vi "Pre-Process Module.vi"(5 "Start Acquire?":bool=TRUE, 6 "Action":string, 7 "Save":bool, 8 "error in":errorcluster, 9 "#pixels to save":i32=200, 10 "start pixel":i32, 11 "#A-lines per B-line":i32=2048) -> (0 "Error Out":errorcluster, 1 "Exit?":bool, 2 "# elements in data queue":i32)   [LabVIEW 2018]
uses:
  Controls/Queue Manager Actions.ctl
  Controls/QueueNames.ctl
  Controls/MessagePacket.ctl
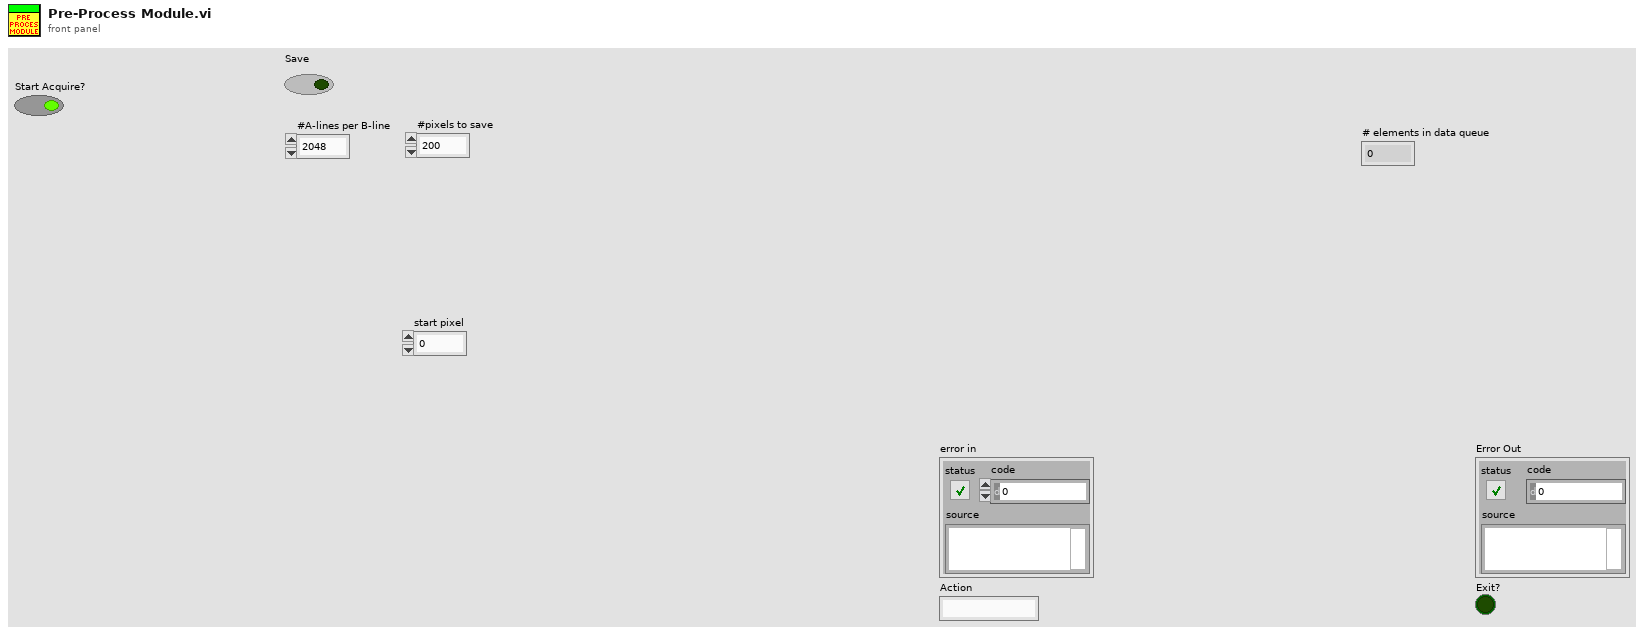
[diagram p1: front panel]
types:
  T1 = typedef "Queue Manager Actions.ctl" = enum16{"Init", "Enqueue", "Enqueue All", "Preview Queue", "Dequeue", "Get Status", "Flush Queue", "Flush All Queues", "Release All Queues", "Release Queue", "Enqueue at Opposite End"}
  T2 = typedef "MessagePacket.ctl" = cluster{"Message":string, "Parameter":variant}
  T3 = typedef "QueueNames.ctl" = enum16{"Main GUI", "Main Scan Processor", "Main Processing", "Main Saving", "Main Display", "Main Table Stage GUI", "Main Table Stage Proc.", "Scan Engine", "Vibratome GUI", "Vibratome Processor", "Slice Engine"}
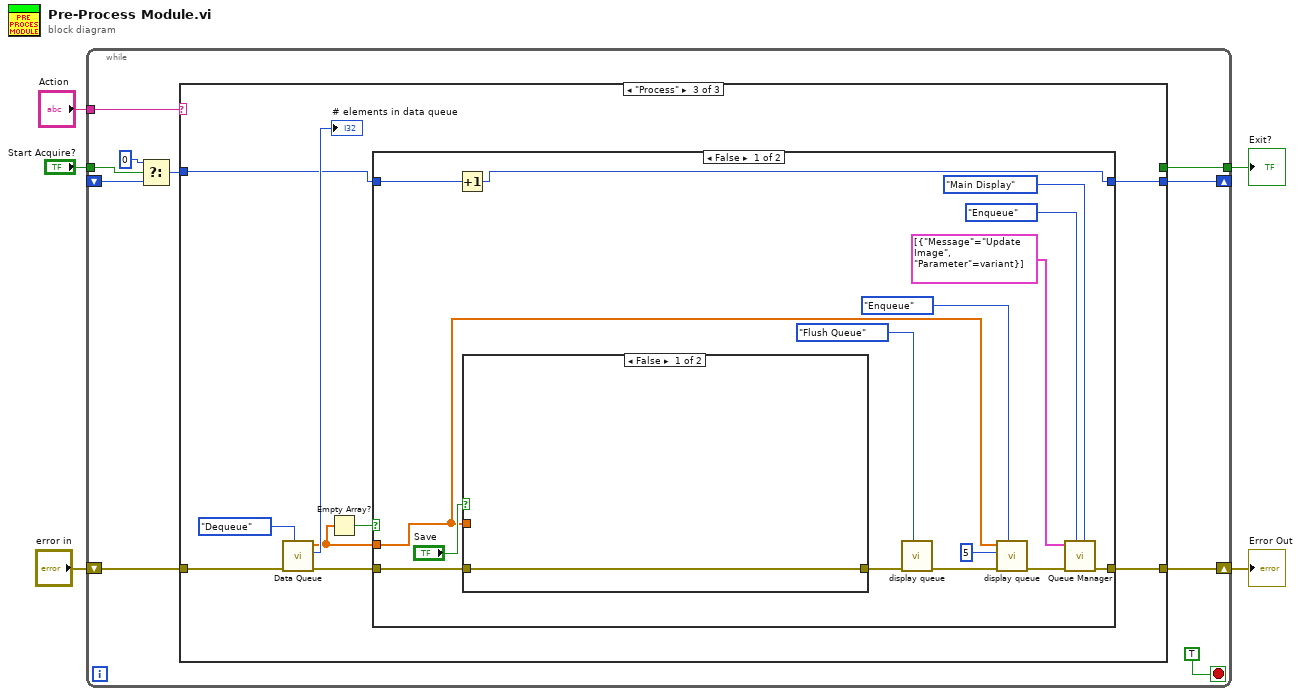
[diagram p0: block diagram]
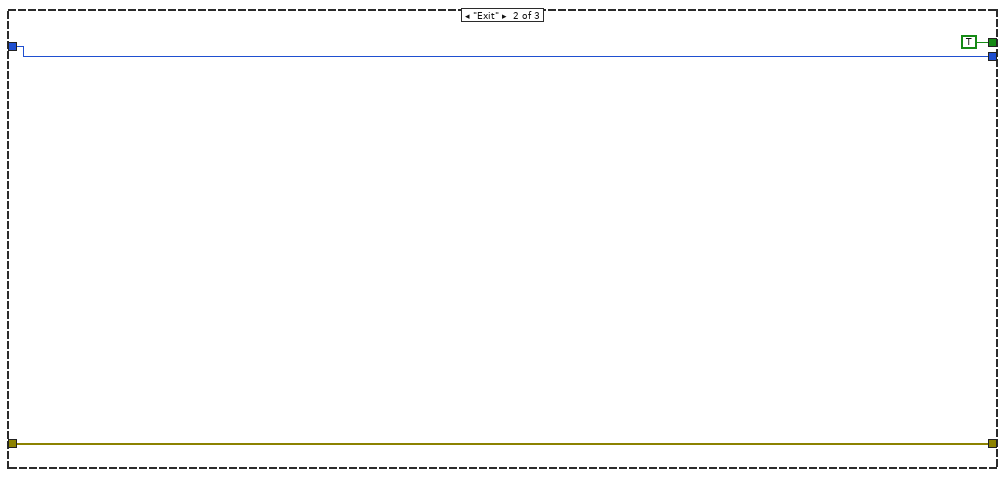
[diagram p3: hidden frame]
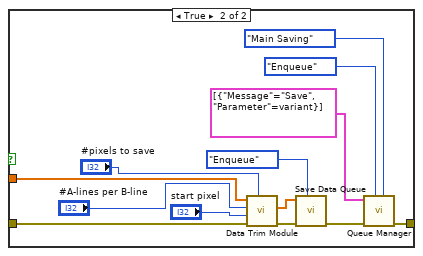
[diagram p4: hidden frame]
diagram:
  n1 = while {
    tunnel: "Action" -> [w13]
    shift-right: [w14] -> w4
    shift-left: "error in" -> [w15]
    tunnel: [w11] -> w2
    shift-right: [w10] -> _
    shift-left: _ -> [w7]
    tunnel: "Start Acquire?" -> [w9]
    stop <- TRUE stop-if-true
    n2 = Select(t=u32 0, s=w9, f=w7) -> (s? t:f=w6:u32)
    n3 = case shown="\"Process\"" w13 {
      tunnel: w15 -> [w17 w19 w28]
      tunnel: [w17 w19 w23] -> w14
      tunnel: [_ TRUE _] -> w11
      tunnel: w6 -> [w16 w18 w22]
      tunnel: [w16 w18 w21] -> w10
      frame "Init", Default {
      }
      frame "Exit" {
      }
      frame "Process" {
        n4 = call "Data Queue.vi"("Action"=Queue_Manager_Actions."Dequeue", "error in (no error)"=w28) -> ("error out"=w26:errorcluster, "# elements in queue"=→"# elements in data queue":i32, "data out"=w24:sgl[])  [unwired: 6 in, 1 out]
        n5 = Empty Array?(array=w24) -> (empty?=w25:bool)
        n6 = case shown="False" w25 {
          tunnel: w26 -> [w41 w60]
          tunnel: [w36 w60] -> w23
          tunnel: w24 -> [w35 _]
          tunnel: [w30 w59] -> w21
          tunnel: w22 -> [w31 w59]
          frame False {
            n7 = Increment(x=w31) -> (x+1=w30:u32)
            n8 = case shown="False" "Save" {
              tunnel: [w45 w53] -> w33
              tunnel: w41 -> [w45 w48]
              tunnel: w35 -> [_ w46]
              frame False {
              }
              frame True {
                n9 = call "Data Trim Module.vi"("#pixels to save"="#pixels to save", "error in"=w48, "start pixel"="start pixel", "#A-lines"="#A-lines per B-line", "1D Array in"=w46) -> ("error out"=w52:errorcluster, "array for saving"=w47:sgl[])  [unwired: 4 in, 1 out]
                n10 = call "Save Data Queue.vi"("Action"=Queue_Manager_Actions."Enqueue", "error in (no error)"=w52, "data in"=w47) -> ("error out"=w54:errorcluster)  [unwired: 5 in, 3 out]
                n11 = call "Queue Manager.vi"("Queue Name"=QueueNames."Main Saving", "Action"=Queue_Manager_Actions."Enqueue", "Error In"=w54, "Message Packet Array"=T2[] [{"Message"="Save", "Parameter"=variant}]) -> ("Error Out"=w53:errorcluster)  [unwired: 3 in, 4 out]
              }
            }
            n12 = call "display queue.vi"("Action"=Queue_Manager_Actions."Flush Queue", "error in (no error)"=w33) -> ("error out"=w34:errorcluster)  [unwired: 5 in, 4 out]
            n13 = call "display queue.vi"("Action"=Queue_Manager_Actions."Enqueue", "error in (no error)"=w34, "time out"=5, "input data"=w35) -> ("error out"=w37:errorcluster)  [unwired: 3 in, 4 out]
            n14 = call "Queue Manager.vi"("Queue Name"=QueueNames."Main Display", "Action"=Queue_Manager_Actions."Enqueue", "Error In"=w37, "Message Packet Array"=T2[] [{"Message"="Update Image", "Parameter"=variant}]) -> ("Error Out"=w36:errorcluster)  [unwired: 3 in, 4 out]
          }
          frame True {
          }
        }
      }
    }
  }
  "Error Out" <- w4
  "Exit?" <- w2
